vi "Random-Graph(real-time).vi"() -> ()   [LabVIEW 2014]
panel:
  out "Waveform Graph":dbl[](graph)
  in  "stop":bool
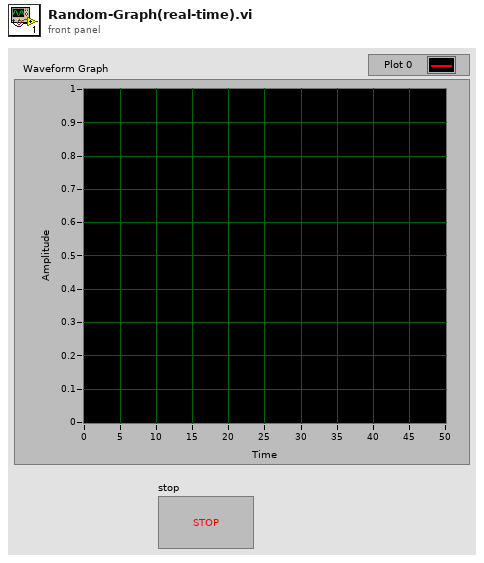
[diagram p1: front panel]
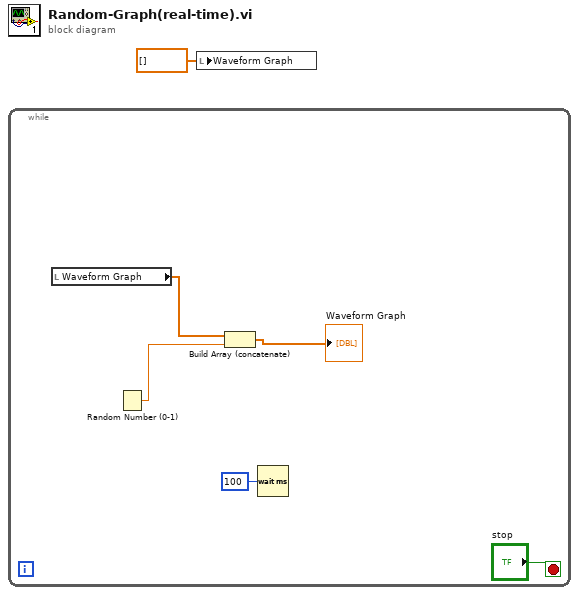
[diagram p0: block diagram]
diagram:
  n1 = while {
    stop <- "stop" stop-if-true
    n2 = local read "Waveform Graph"() -> (w5:dbl[])
    n3 = Random Number (0-1)() -> (number: 0 to 1=w4:dbl)
    n4 = Build Array (concatenate)(w5, w4) -> (→"Waveform Graph":dbl[])
    n5 = Wait (ms)(milliseconds to wait=u32 100) -> ()  [unwired: 1 out]
  }
  n6 = local write "Waveform Graph"(dbl[] [] ("Waveform Graph")) -> ()
